vi "Mercury_GCS_Sample_Application_DaisyChain.vi"(11 "error in":errorcluster) -> (15 "error out":errorcluster)   [LabVIEW 2012]
doc: "This VI demonstrates how to define a Mercury DaisyChain configuration with two Mercury controllers (with GCS firmware) in the chain and stages connected. In this example, the first Mercury is connected through COM port 1 with baudrate 38400. The VI runs Mercury_GCS_Configuration_Setup.vi for both controllers with pre-defined settings and reads the position of the axes. The diagram shows how to combine the driver VIs for these tasks.\nWarning: This VI has Interface settings for the first controller in the chain that probably do not match your current configuration. Please modify the \"Interface\", \"RS232 settings\" or \"USB settings\" in the diagram before running the VI. All controllers in the chain must use the same baudrate (which can be set with the DIP switches on the Mercury front panel)."
panel:
  in  "stop":bool
  out "Position system 2":dbl[](array[numeric]) format="%.6f"
  out "Identification Mercury controller 2":string
  out "Conn. Axes system 2":string[](array[string])
  out "Running":bool caption="Mercury_GCS_Configuration_Setup.vi is running"
  out "Position system 1":dbl[](array[numeric]) format="%.6f"
  out "Conn. Axes system 1":string[](array[string])
  out "Identification Mercury controller 1":string
  # "Simple Mercury GCS sample program (two systems, connection\nvia DaisyChain)"
  # "This VI demonstrates how to define a Mercury DaisyChain configuration with two Mercury controllers (with GCS firmware)  in the chain and stages \nconnected. In this example, the first Mercury is connected through COM port 1 with baudrate 38400. The VI runs Mercury_GCS_Configuration_Setup.vi \nfor both controllers with pre-defined settings and reads the position of the axes. The diagram shows how to combine the driver VIs for these tasks.\n\nWarning: This VI has Interface settings for the first controller in the chain that probably do not match your current configuration. \n                 Please modify the \"Interface\", \"RS232 settings\" or \"USB settings\" in the diagram before running the VI. All controllers in the \n                 chain must use the same baudrate (which can be set with the DIP switches on the Mercury front panel)."
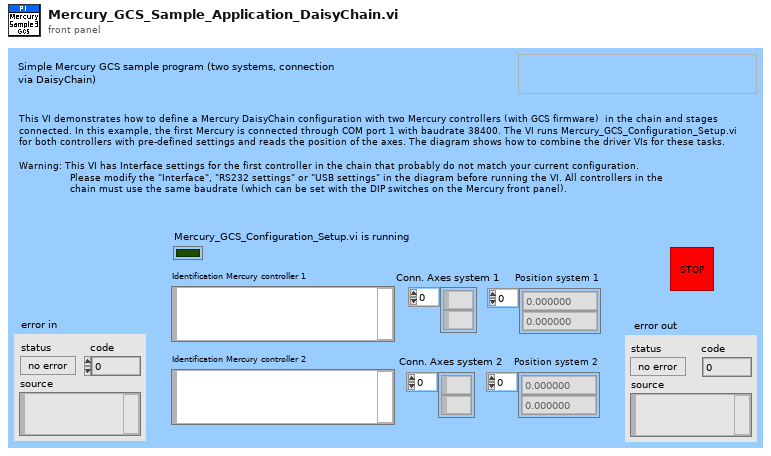
[diagram p1: front panel]
types:
  T1 = cluster{"Register DC":bool, "DaisyChain Search?":bool, "Device ID":i32}
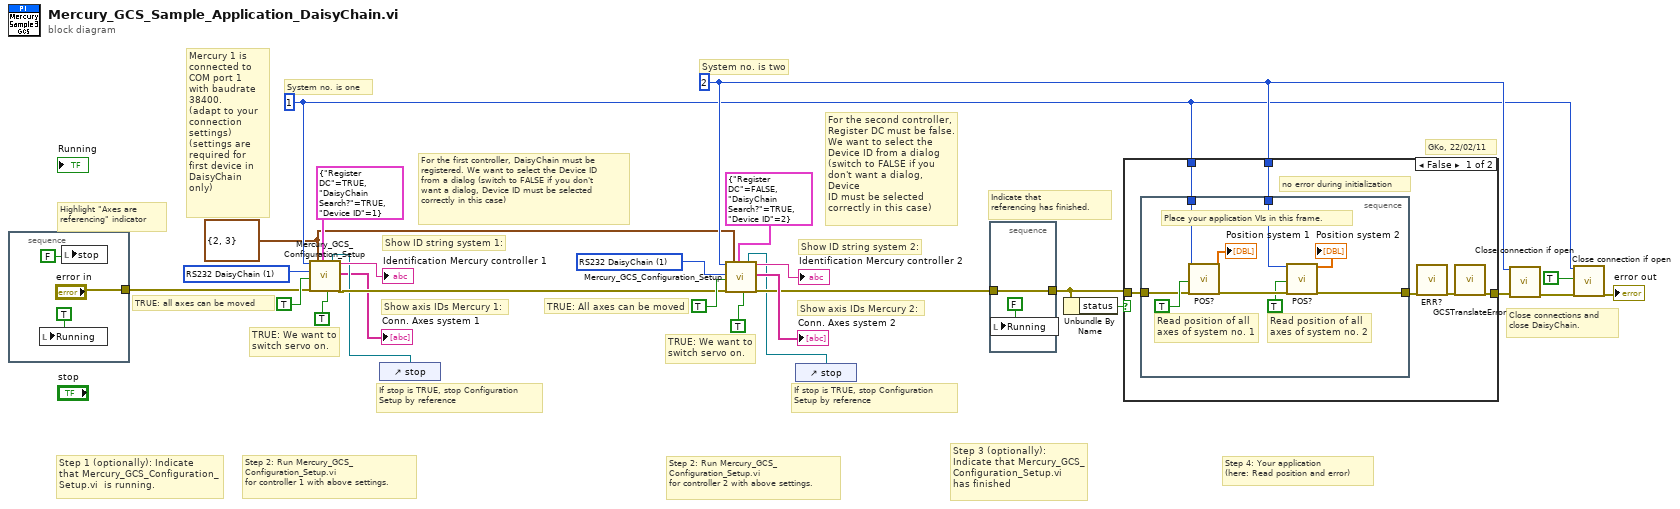
[diagram p0: block diagram]
diagram:
  w1 = u16 1 items=["RS232", "RS232 DaisyChain", "USB", "USB_DaisyChain"] ("Interface")
  w2 = u16 1 items=["RS232", "RS232 DaisyChain", "USB", "USB_DaisyChain"] ("Interface")
  w3 = cluster{"Portnumber":i32, "Baudrate":u16} {"Portnumber"=2, "Baudrate"=3} ("RS232 settings")
  w7 = 2 ("System no.")
  w6 = 1 ("System no.")
  # "Close connections and\nclose DaisyChain."
  # "For the second controller,\nRegister DC must be false.\nWe want to select the \nDevice ID from a dialog \n(switch to FALSE if you \ndon't want a dialog, Device\nID must be selected\ncorrectly in this case)"
  # "Step 4: Your application\n(here: Read position and error)"
  # "For the first controller, DaisyChain must be\nregistered. We want to select the Device ID\nfrom a dialog (switch to FALSE if you don't\nwant a dialog, Device ID must be selected\ncorrectly in this case)"
  # "Mercury 1 is\nconnected to\nCOM port 1\nwith baudrate\n38400.\n(adapt to your\nconnection\nsettings)\n(settings are\nrequired for \nfirst device in\nDaisyChain only)"
  # "If stop is TRUE, stop Configuration\nSetup by reference"
  # "If stop is TRUE, stop Configuration\nSetup by reference"
  # "Step 2: Run Mercury_GCS_\nConfiguration_Setup.vi\nfor controller 2 with above settings."
  # "Show axis IDs Mercury 2:"
  # "Show ID string system 2:"
  # "TRUE: We want to\nswitch servo on."
  # "TRUE: All axes can be moved"
  # "System no. is two"
  # "GKo, 22/02/11"
  # "Step 3 (optionally): \nIndicate that Mercury_GCS_\nConfiguration_Setup.vi\nhas finished"
  # "Step 2: Run Mercury_GCS_\nConfiguration_Setup.vi\nfor controller 1 with above settings."
  # "Step 1 (optionally): Indicate\nthat Mercury_GCS_Configuration_\nSetup.vi  is running."
  # "Indicate that\nreferencing has finished."
  # "Highlight \"Axes are\nreferencing\" indicator"
  # "Show axis IDs Mercury 1:"
  # "Show ID string system 1:"
  # "TRUE: We want to\nswitch servo on."
  # "TRUE: all axes can be moved"
  # "System no. is one"
  n1 = stacked-sequence {
    tunnel: ["error in"] -> w23
    frame #0 {
      n2 = local write "Running"(TRUE ("Running")) -> ()
      n3 = local write "stop"(FALSE ("stop")) -> ()
    }
  }
  n4 = control-ref of="stop"() -> (w16:refnum<vi>)
  n5 = call "Mercury_GCS_Configuration_Setup.vi"("System no."=w6, "Interface"=w2, "All axes?"=TRUE, "error in"=w23, "RS232 settings"=w3, "DaisyChain settings"=T1 {"Register DC"=TRUE, "DaisyChain Search?"=TRUE, "Device ID"=1} ("RS232 DaisyChain settings"), "Switch servo on?"=TRUE ("Use dialog to define\nconnected stages?"), "Stop refnum"=w16) -> ("Identification"=→"Identification Mercury controller 1":string, "Conn. \nAxes"=→"Conn. Axes system 1":string[], "error out"=w18:errorcluster)  [unwired: 5 in, 4 out]
  n6 = control-ref of="stop"() -> (w15:refnum<vi>)
  n7 = call "Mercury_GCS_Configuration_Setup.vi"("System no."=w7, "Interface"=w1, "All axes?"=TRUE, "error in"=w18, "RS232 settings"=w3, "DaisyChain settings"=T1 {"Register DC"=FALSE, "DaisyChain Search?"=TRUE, "Device ID"=2} ("RS232 DaisyChain settings"), "Switch servo on?"=TRUE ("Use dialog to define\nconnected stages?"), "Stop refnum"=w15) -> ("Identification"=→"Identification Mercury controller 2":string, "Conn. \nAxes"=→"Conn. Axes system 2":string[], "error out"=w17:errorcluster)  [unwired: 5 in, 4 out]
  n8 = stacked-sequence {
    tunnel: w17 -> [w31]
    tunnel: [w31] -> w12
    frame #0 {
      n9 = local write "Running"(FALSE ("Running")) -> ()
    }
  }
  n10 = Unbundle By Name(w12) -> ("status"=w13:bool)
  n11 = case shown="False" w13 {
    tunnel: w6 -> [w37 _]
    tunnel: w12 -> [w36 w47]
    tunnel: [w33 w47] -> w11
    tunnel: w7 -> [w32 _]
    frame False {
      # "no error during initialization"
      n12 = stacked-sequence {
        tunnel: w37 -> [w46]
        tunnel: [w40] -> w34
        tunnel: w36 -> [w44]
        tunnel: w32 -> [w38]
        frame #0 {
          # "Read position of all\naxes of system no. 2"
          # "Read position of all \naxes of system no. 1"
          # "Place your application VIs in this frame."
          n13 = call "POS?.vi"("System no."=w46, "All axes?"=TRUE, "error in"=w44) -> ("Position"=→"Position system 1":dbl[], "error out"=w41:errorcluster)  [unwired: 15 in]
          n14 = call "POS?.vi"("System no."=w38, "All axes?"=TRUE, "error in"=w41) -> ("Position"=→"Position system 2":dbl[], "error out"=w40:errorcluster)  [unwired: 15 in]
        }
      }
      n15 = call "ERR?.vi"("error in"=w34) -> ("error out"=w35:errorcluster)  [unwired: 17 in, 1 out]
      n16 = call "GCSTranslateError.vi"("error in"=w35) -> ("error out"=w33:errorcluster)  [unwired: 16 in, 2 out]
    }
    frame True {
      # "error during initialization!"
    }
  }
  n17 = call "Close connection if open.vi"("System no."=w7, "error in"=w11) -> ("error out"=w10:errorcluster)  [unwired: 16 in, 1 out]
  n18 = call "Close connection if open.vi"("System no."=w6, "Close DaisyChain"=TRUE, "error in"=w10) -> ("error out"=→"error out":errorcluster)  [unwired: 15 in, 1 out]
